vi "Simple.vi"() -> ()   [LabVIEW 2017]
doc: "Shows how to alphabetize cluster controls, indicators, and constants that are arranged vertically or horizontally using the Shortcut Menu Plugin (SMP) and/or the Quick-Drop Keyboard Shortcut (QDKS). It is NOT required for the clusters to be arranged vertically or horizontally, but it is recommended."
panel:
  out "Cluster 4":T1
  out "Cluster 3":T1
  in  "Cluster 2":T1
  in  "Cluster 1":T1
  # "Overview: Demonstrates alphabetizing clusters using the Shortcut Menu Plug-in (SMP) and the Quick Drop Keyboard Shortcut (QDKS)\nInstructions:\n1. Right-click on the border of a cluster control\n2. Select Alphabetize from the Shortcut Menu that appears \n3. Select another un-alphabetized cluster.\n4. Display the Quick Drop dialog with CTRL+SPACE\n5. Use the alphabetize shortcut of CTRL+C\n7. Switch to the block diagram\n8. Repeat steps 1-5 for the cluster constants instead of the cluster controls."
  # "Note, each cluster is arranged either vertically or horizontally but this is not a requirement."
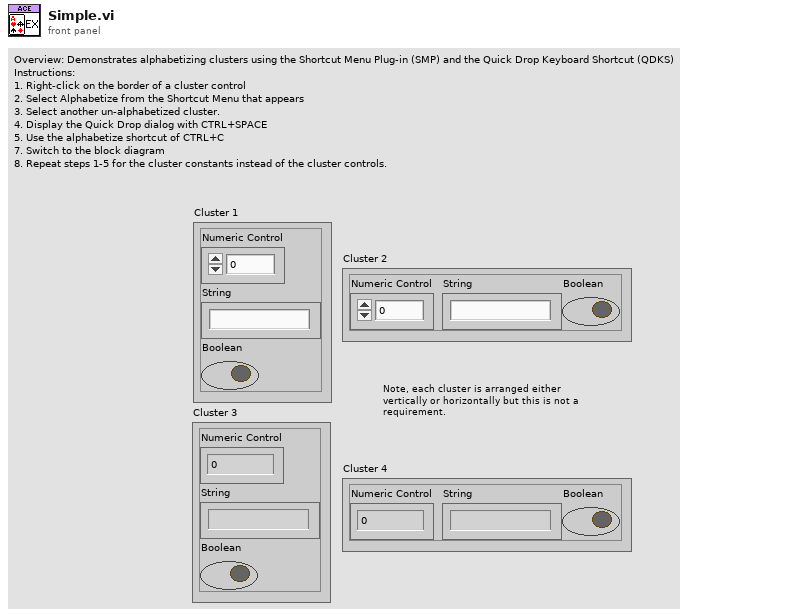
[diagram p1: front panel]
types:
  T1 = cluster{"Numeric Control":dbl, "String":string, "Boolean":bool}
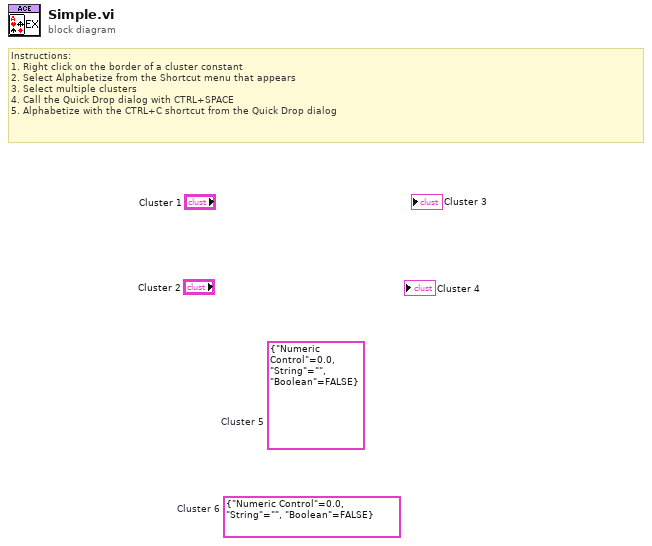
[diagram p0: block diagram]
diagram:
  (unwired) T1 {"Numeric Control"=0.0, "String"="", "Boolean"=FALSE}  # Cluster 6
  (unwired) T1 {"Numeric Control"=0.0, "String"="", "Boolean"=FALSE}  # Cluster 5
  # "Instructions:\n1. Right click on the border of a cluster constant \n2. Select Alphabetize from the Shortcut menu that appears\n3. Select multiple clusters\n4. Call the Quick Drop dialog with CTRL+SPACE\n5. Alphabetize with the CTRL+C shortcut from the Quick Drop dialog"
